vi "PH_Beckhoff.scale analog DIM Value.vi"(0 "DIM value":dbl, 1 "Sca Type":u32) -> (2 "Beckhoff value":u32)   [LabVIEW 2014, in "PH_Beckhoff.lvlib"]
doc: "This VI is forseen to scale the DIM value to the raw digital Beckhoff value to be set."
uses:
  PH_Beckhoff.lvlib
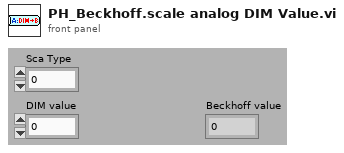
[diagram p1: front panel]
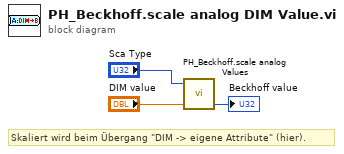
[diagram p0: block diagram]
diagram:
  # "Skaliert wird beim Übergang \"DIM -> eigene Attribute\" (hier)."
  n1 = call "PH_Beckhoff.scale analog Values.vi"("DIM value"="DIM value", "Sca Type"="Sca Type") -> ("Scaled Beckhoff value"=→"Beckhoff value":u32)  [unwired: 1 in, 2 out]
